vi "Zaber A Series XYZ List.vi"() -> ()   [LabVIEW 2013]
doc: "This example moves a system of up to three axes through a list of co-ordinates. It uses the Move command as well as the Poll Until Idle library VI to co-ordinate the timing of the movements of the stages."
uses:
  Zaber A Series.lvlib
  <vilib>/Utility/file.llb/Read Delimited Spreadsheet (string).vi
panel:
  in  "Read Coordinates from CSV":path
  in  "Z-Axis Microstep Size (0)":dbl
  in  "Z Device and Axis (03)":string="03"
  in  "Units (0: microsteps)":u16(ring) items=["microsteps", "microns", "millimeters", "inches"]
  in  "Movement Type (0: relative)":u16(ring) items=["relative", "absolute"]
  in  "Y-Axis Microstep Size (0)":dbl
  in  "XYZ Positions":string[][](table)
  in  "Y Device and Axis (02)":string="02"
  in  "X Device and Axis (01)":string="01"
  in  "X-Axis Microstep Size (0)":dbl
  in  "VISA resource name":refnum<visa-resource-name>
  # "(c) 2017 Zaber Technologies.  ALL RIGHTS RESERVED."
  # "This example demonstrates how you can move between co-ordinates. Before running, enter all of the XYZ points you'd like your stages to move to and the VISA resource name of your conenction. Make sure the units of your positions match the units dropdown. Also ensure that the Axis numbers correspond to your device numbers. Finally enter the microstep sizes of the devices if you are using something other than microsteps.\n\nEnter a file path in the Read Coordinates from CSV field if you'd like to use a spreadsheet to load the points.\n\nThis example can be used for one or two axes only by omitting coordinates. Only non-empty fields will be read."
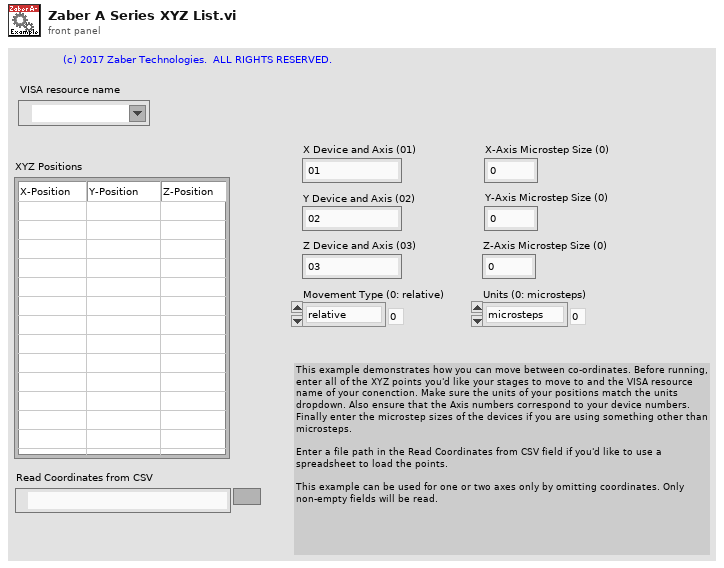
[diagram p1: front panel]
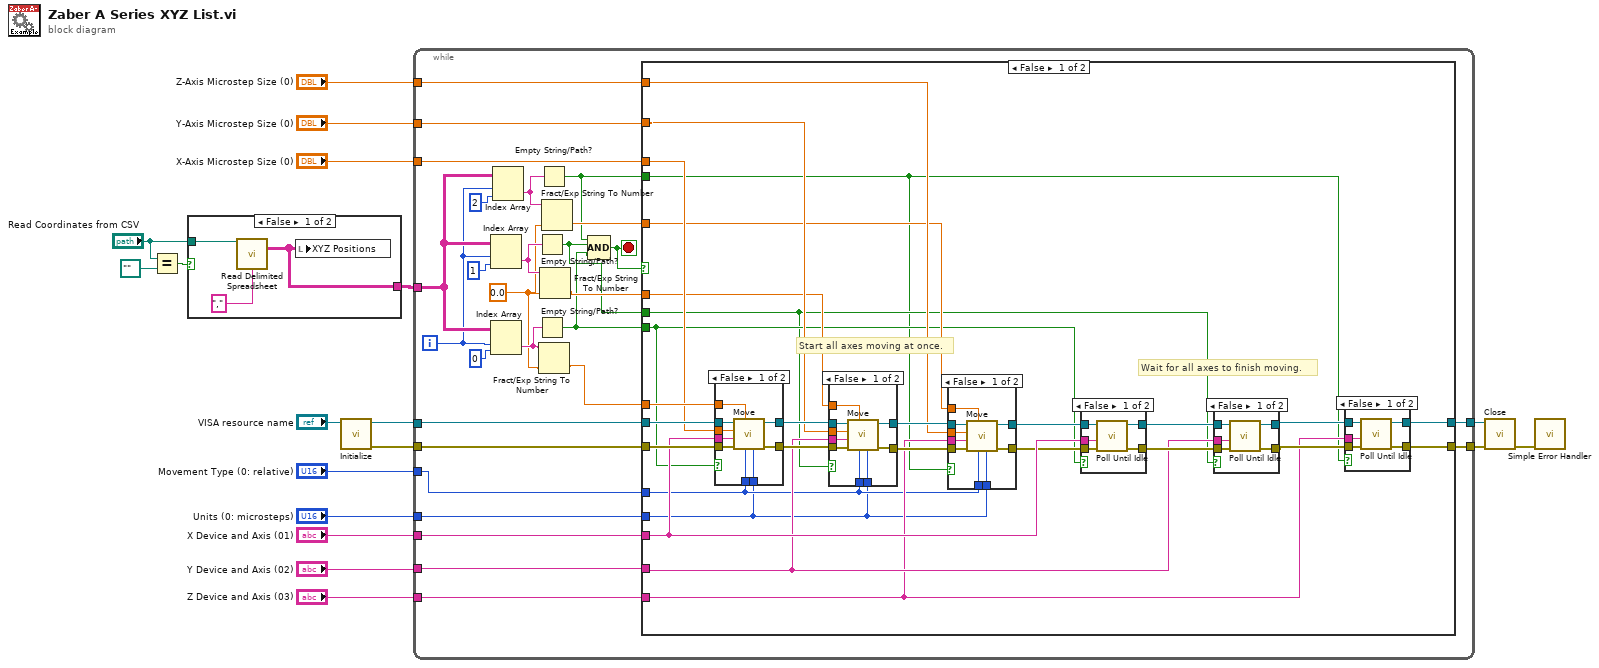
[diagram p0: block diagram]
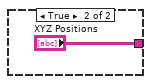
[diagram p2: hidden frame]
diagram:
  n1 = Equal?(x="Read Coordinates from CSV", y=path "") -> (x = y?=w1:bool)
  n2 = case shown="False" w1 {
    tunnel: "Read Coordinates from CSV" -> [w20 _]
    tunnel: [w19 "XYZ Positions"] -> w4
    frame False {
      n3 = call-poly <vilib>:"Read Delimited Spreadsheet.vi"("file path (dialog if empty)"=w20, "delimiter (\\t)"="," ("delimiter (\\t)")) -> ("all rows"=w19:string[][])  [unwired: 8 in, 5 out]
      n4 = local write "XYZ Positions"(w19) -> ()
    }
    frame True {
    }
  }
  n5 = call "Initialize.vi"("VISA resource name"="VISA resource name") -> ("error out"=w12:errorcluster, "VISA resource name out"=w17:refnum<visa-resource-name>)  [unwired: 9 in]
  n6 = while {
    tunnel: w17 -> [w50]
    tunnel: w4 -> [w31]
    tunnel: "Units (0: microsteps)" -> [w47]
    tunnel: "Movement Type (0: relative)" -> [w46]
    tunnel: "Y Device and Axis (02)" -> [w45]
    tunnel: "X Device and Axis (01)" -> [w44]
    tunnel: w12 -> [w43]
    tunnel: [w42] -> w11
    tunnel: [w41] -> w10
    tunnel: "Y-Axis Microstep Size (0)" -> [w40]
    tunnel: "X-Axis Microstep Size (0)" -> [w39]
    tunnel: "Z Device and Axis (03)" -> [w34]
    tunnel: "Z-Axis Microstep Size (0)" -> [w33]
    i -> [w30]
    stop <- w26 stop-if-true
    w29 = 0.0
    n7 = Index Array(array=w31, index (row)=w30, index (col)=1 ("disabled index (col)")) -> (element=w38:string)
    n8 = Index Array(array=w31, index (row)=w30, index (col)=0 ("disabled index (col)")) -> (element=w35:string)
    n9 = Index Array(array=w31, index (row)=w30, index (col)=2 ("disabled index (col)")) -> (element=w27:string)
    n10 = Empty String/Path?(string/path=w38) -> (empty?=w23:bool)
    n11 = Empty String/Path?(string/path=w35) -> (empty?=w24:bool)
    n12 = Empty String/Path?(string/path=w27) -> (empty?=w25:bool)
    n13 = Fract/Exp String To Number(string=w35, default (0 dbl)=w29) -> (number=w36:dbl)  [unwired: 2 in, 1 out]
    n14 = Fract/Exp String To Number(string=w38, default (0 dbl)=w29) -> (number=w37:dbl)  [unwired: 2 in, 1 out]
    n15 = Fract/Exp String To Number(string=w27, default (0 dbl)=w29) -> (number=w28:dbl)  [unwired: 2 in, 1 out]
    n16 = Compound Arithmetic op=AND(w25, w23, w24) -> (w26:bool)
    n17 = case shown="False" w26 {
      tunnel: w47 -> [w58 _]
      tunnel: w50 -> [w77 w133]
      tunnel: w44 -> [w68 _]
      tunnel: w45 -> [w61 _]
      tunnel: w46 -> [w59 _]
      tunnel: w36 -> [w78 _]
      tunnel: w37 -> [w55 _]
      tunnel: w43 -> [w76 w134]
      tunnel: [w73 w134] -> w41
      tunnel: [w74 w133] -> w42
      tunnel: w40 -> [w57 _]
      tunnel: w39 -> [w75 _]
      tunnel: w34 -> [w60 _]
      tunnel: w33 -> [w56 _]
      tunnel: w28 -> [w54 _]
      tunnel: w25 -> [w51 _]
      tunnel: w24 -> [w53 _]
      tunnel: w23 -> [w52 _]
      frame False {
        # "Start all axes moving at once."
        # "Wait for all axes to finish moving."
        n18 = case shown="False" w53 {
          tunnel: w58 -> [w109 _]
          tunnel: [w108 w111] -> w67
          tunnel: w59 -> [w107 _]
          tunnel: w78 -> [w106 _]
          tunnel: w77 -> [w105 w111]
          tunnel: w76 -> [w104 w110]
          tunnel: [w103 w110] -> w66
          tunnel: w75 -> [w102 _]
          tunnel: w68 -> [w101 _]
          frame False {
            n19 = call "Move.vi"("Units (0: microsteps)"=w109, "Movement Type (0: relative)"=w107, "Move Distance (0)"=w106, "error in (no error)"=w104, "Device and Axis"=w101, "Microstep Size (0)"=w102, "VISA resource name"=w105) -> ("error out"=w103:errorcluster, "VISA resource name out"=w108:refnum<visa-resource-name>)  [unwired: 3 in]
          }
          frame True {
          }
        }
        n20 = case shown="False" w52 {
          tunnel: w58 -> [w98 _]
          tunnel: [w97 w100] -> w65
          tunnel: w59 -> [w96 _]
          tunnel: w55 -> [w95 _]
          tunnel: w67 -> [w94 w100]
          tunnel: w66 -> [w91 w99]
          tunnel: [w90 w99] -> w64
          tunnel: w57 -> [w93 _]
          tunnel: w61 -> [w92 _]
          frame False {
            n21 = call "Move.vi"("Units (0: microsteps)"=w98, "Movement Type (0: relative)"=w96, "Move Distance (0)"=w95, "error in (no error)"=w91, "Device and Axis"=w92, "Microstep Size (0)"=w93, "VISA resource name"=w94) -> ("error out"=w90:errorcluster, "VISA resource name out"=w97:refnum<visa-resource-name>)  [unwired: 3 in]
          }
          frame True {
          }
        }
        n22 = case shown="False" w51 {
          tunnel: w58 -> [w87 _]
          tunnel: [w86 w89] -> w63
          tunnel: w59 -> [w85 _]
          tunnel: w54 -> [w84 _]
          tunnel: w65 -> [w83 w89]
          tunnel: w64 -> [w82 w88]
          tunnel: [w81 w88] -> w62
          tunnel: w56 -> [w80 _]
          tunnel: w60 -> [w79 _]
          frame False {
            n23 = call "Move.vi"("Units (0: microsteps)"=w87, "Movement Type (0: relative)"=w85, "Move Distance (0)"=w84, "error in (no error)"=w82, "Device and Axis"=w79, "Microstep Size (0)"=w80, "VISA resource name"=w83) -> ("error out"=w81:errorcluster, "VISA resource name out"=w86:refnum<visa-resource-name>)  [unwired: 3 in]
          }
          frame True {
          }
        }
        n24 = case shown="False" w53 {
          tunnel: w63 -> [w130 w132]
          tunnel: w68 -> [w129 _]
          tunnel: w62 -> [w128 w131]
          tunnel: [w127 w131] -> w69
          tunnel: [w126 w132] -> w70
          frame False {
            n25 = call "Poll Until Idle.vi"("error in (no error)"=w128, "Device and Axis"=w129, "VISA resource name"=w130) -> ("error out"=w127:errorcluster, "VISA resource name out"=w126:refnum<visa-resource-name>)  [unwired: 7 in]
          }
          frame True {
          }
        }
        n26 = case shown="False" w52 {
          tunnel: w70 -> [w123 w125]
          tunnel: w61 -> [w122 _]
          tunnel: w69 -> [w121 w124]
          tunnel: [w120 w124] -> w71
          tunnel: [w119 w125] -> w72
          frame False {
            n27 = call "Poll Until Idle.vi"("error in (no error)"=w121, "Device and Axis"=w122, "VISA resource name"=w123) -> ("error out"=w120:errorcluster, "VISA resource name out"=w119:refnum<visa-resource-name>)  [unwired: 7 in]
          }
          frame True {
          }
        }
        n28 = case shown="False" w51 {
          tunnel: w72 -> [w116 w118]
          tunnel: w60 -> [w115 _]
          tunnel: w71 -> [w114 w117]
          tunnel: [w113 w117] -> w73
          tunnel: [w112 w118] -> w74
          frame False {
            n29 = call "Poll Until Idle.vi"("error in (no error)"=w114, "Device and Axis"=w115, "VISA resource name"=w116) -> ("error out"=w113:errorcluster, "VISA resource name out"=w112:refnum<visa-resource-name>)  [unwired: 7 in]
          }
          frame True {
          }
        }
      }
      frame True {
      }
    }
  }
  n30 = call "Close.vi"("error in (no error)"=w10, "VISA resource name"=w11) -> ("error out"=w9:errorcluster)  [unwired: 9 in]
  n31 = call <vilib>:"Simple Error Handler.vi"("error in (no error)"=w9) -> ()  [unwired: 4 in, 5 out]
